vi "Run Process And Alg.vi"(7 "Process":bool, 8 "error in (no error)":errorcluster, 9 "CheckDist":bool, 10 "ROIList":string[][](array[string]), 11 "Image":T2(plugin-control)) -> (0 "Result Arr":T1(array[cluster]), 1 "DetectOut":variant[](array[variant]), 2 "ALLResultOut":string[][](array[string]), 3 "AlgOut":i32[](array[numeric]), 4 "error out":errorcluster)   [LabVIEW 2019]
uses:
  a08a38d4-8fb3-4640-b0fd-20f744aeac5c.vi
  1e835489-0bb4-467e-a464-32fccfa39e30.vi
  <vilib>/JDP Science/JSONtext/JSON text to Variant.vi
  Main UI/Glb/Main_UI Gb.vi
panel:
  out "x-y":u32
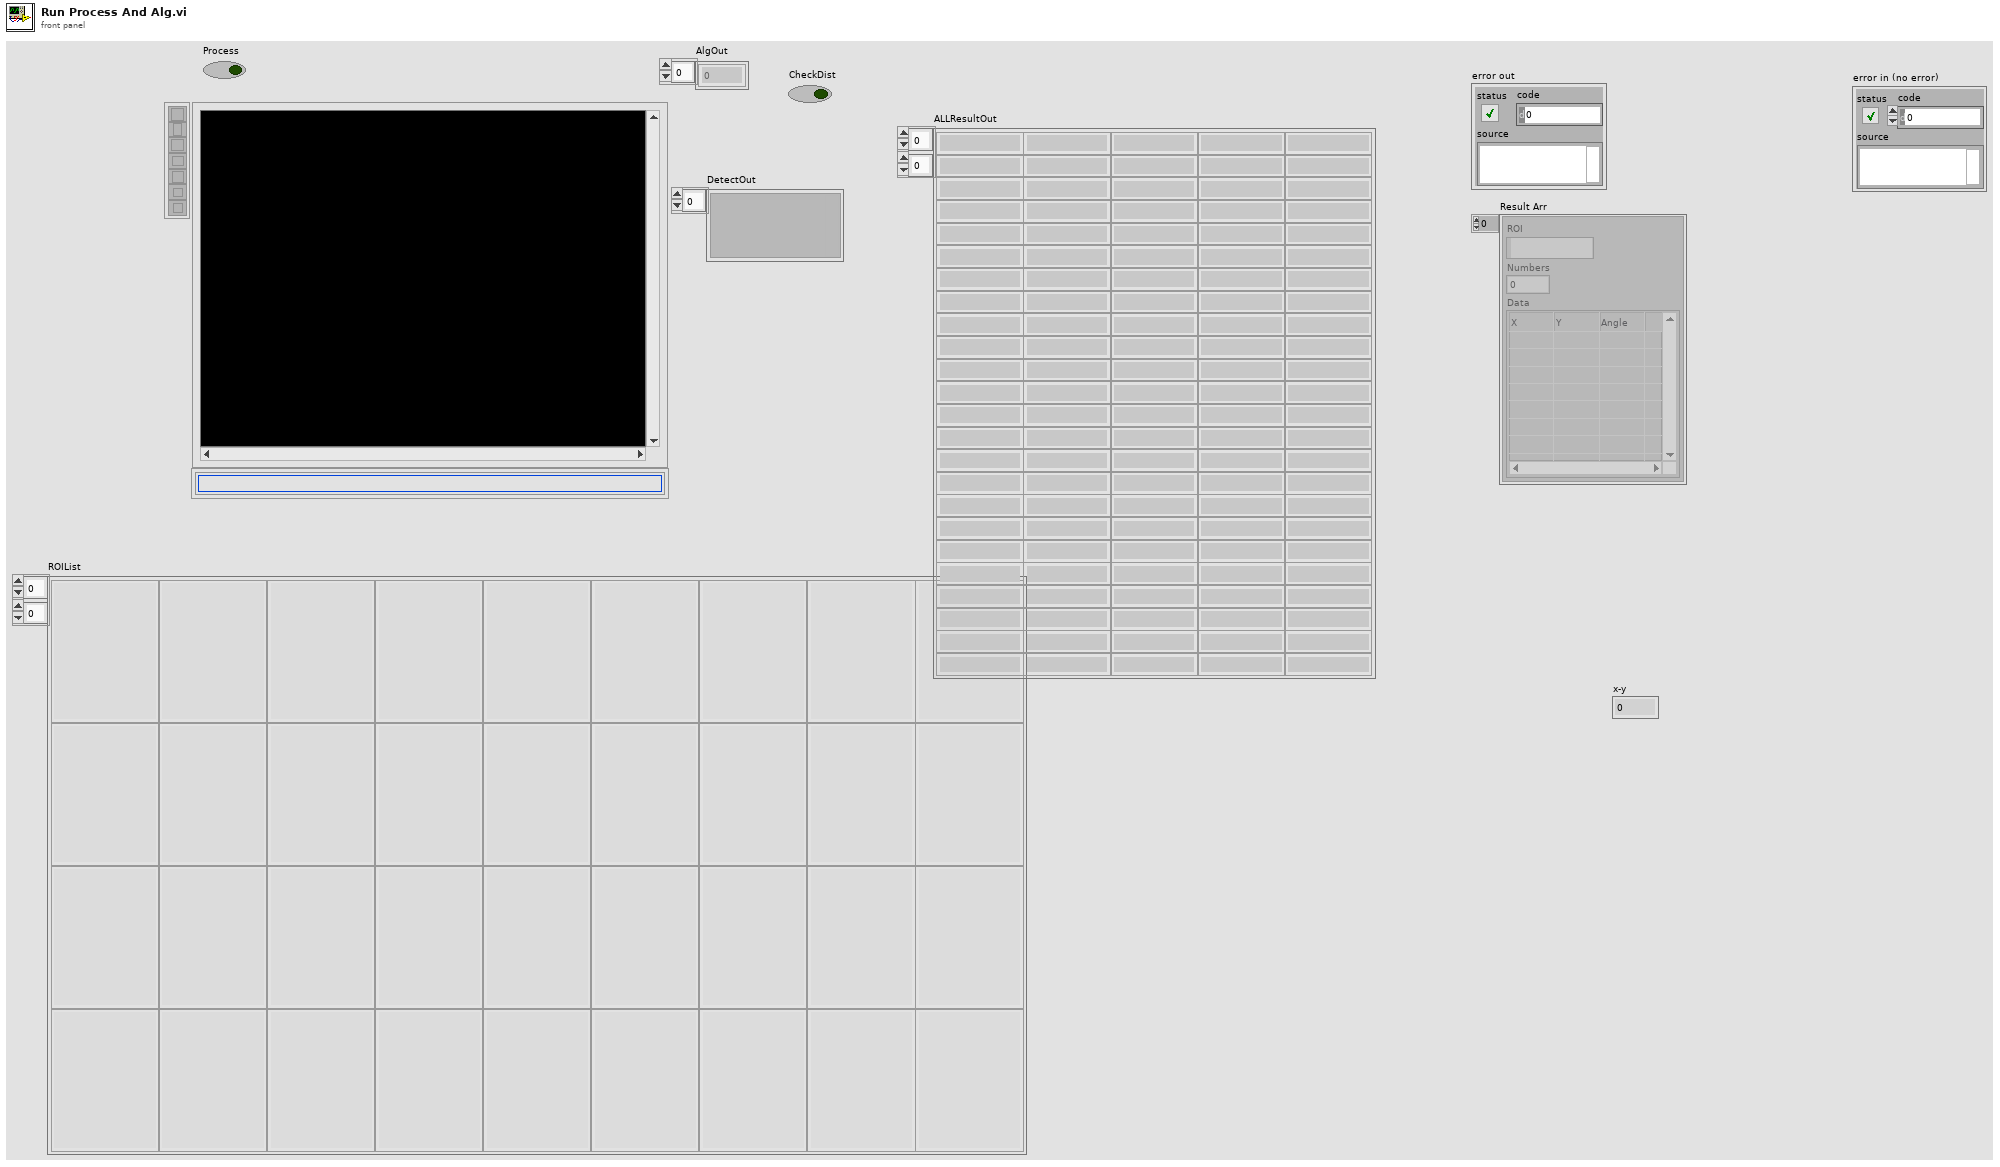
[diagram p1: front panel]
types:
  T1 = cluster{"ROI":string, "Numbers":i32, "Data":string[][]}[]
  T2 = typedef "IMAQ Image.ctl" = refnum<image>
  T3 = enum16{"Init", "Grab", "Get All", "Close", "Set Camera"}
  T4 = typedef "IMAQdx.ctl" = refnum<k21>
  T5 = cluster{"Desired Font (Application)":enum16{"User-specified Font", "Application Font", "System Font", "Dialog Font"}, "[User-specified Font]":cluster{"Font Name":string, "Size":i16, "Strikeout?":bool, "Italic?":bool, "Underline?":bool, "Outline?":bool, "Shadow?":bool, "Bold?":bool, "Rotation Angle":dbl}, "Horizontal Alignment":i16, "Vertical Alignment":i16}
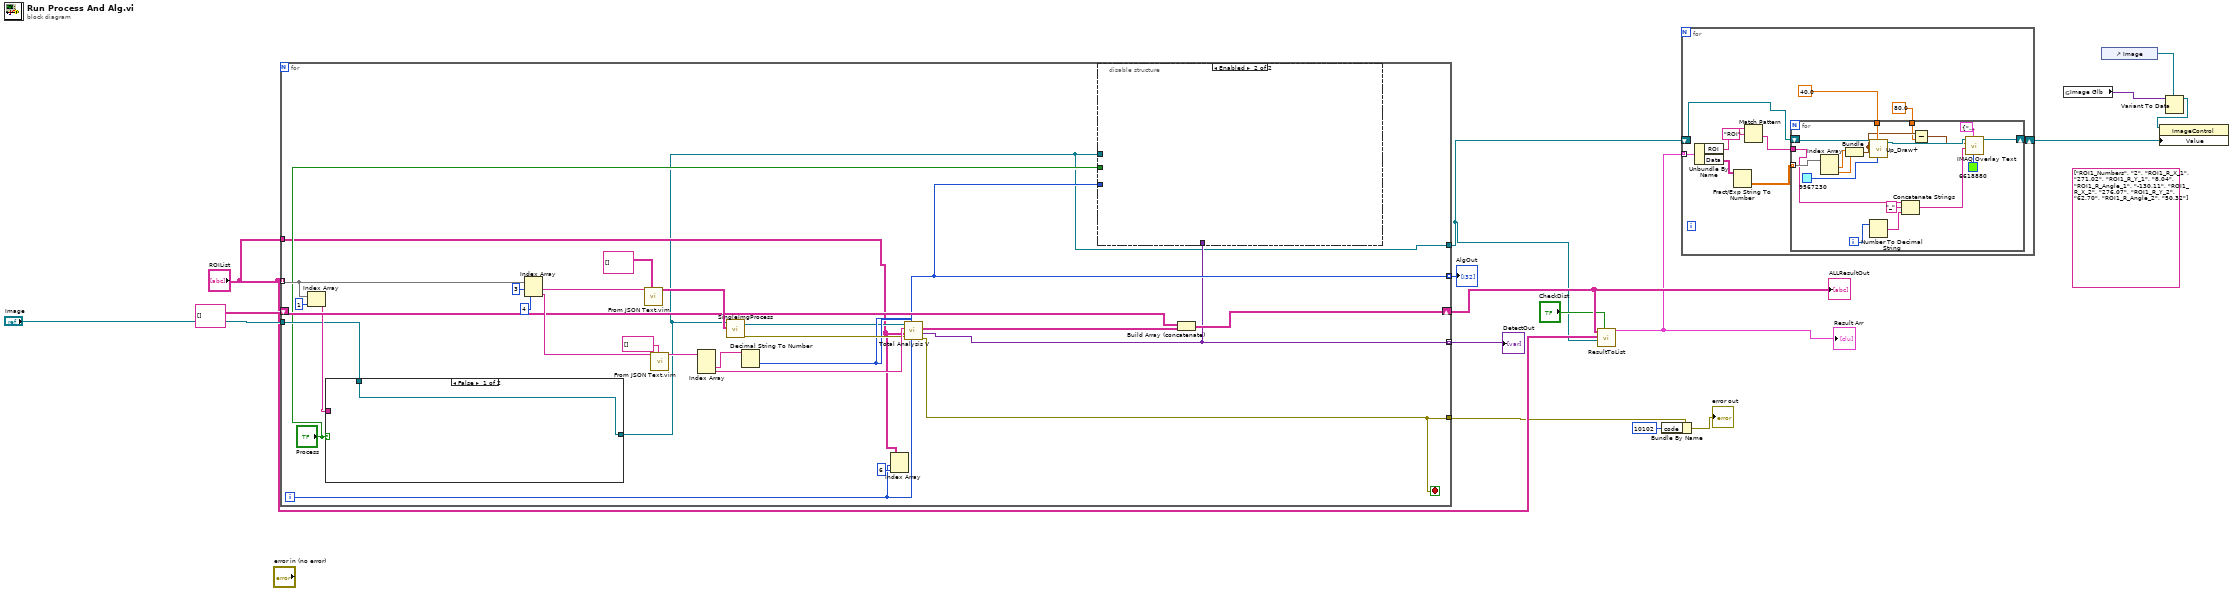
[diagram p0: block diagram]
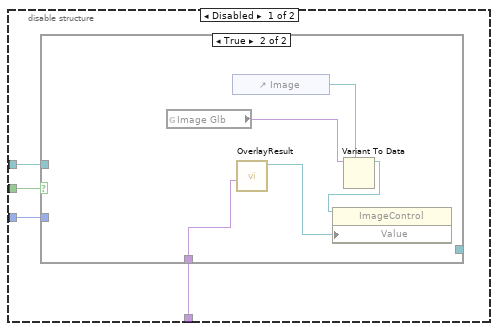
[diagram p2: hidden frame]
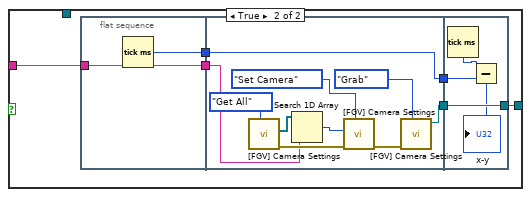
[diagram p4: hidden frame]
diagram:
  (unwired) string[][] [["ROI1_Numbers", "2"], ["ROI1_R_X_1", "271.02"], ["ROI1_R_Y_1", "8.04"], ["ROI1_R_Angle_1", "-130.11"], ["ROI1_R_X_2", "276.07"], ["ROI1_R_Y_2", "62.70"], ["ROI1_R_Angle_2", "50.32"]] ("ResultOut 2")
  n1 = for {
    tunnel: "ROIList" -> [w29] mode=indexing
    tunnel: "Image" -> [w26]
    shift-right: [w33] -> w13
    shift-left: string[][] [] -> [w32]
    tunnel: [w24] -> w3 mode=indexing
    tunnel: [w25] -> w14 mode=indexing
    tunnel: "ROIList" -> [w19]
    tunnel: [w18] -> w6
    tunnel: [w17] -> w1
    i -> [w21]
    stop <- w18 stop-if-true
    n2 = Index Array(array=w29, index=1) -> (element=w27:string)
    n3 = case shown="False" "Process" {
      tunnel: w27 -> [_ w60]
      tunnel: [w54 w59] -> w17
      tunnel: w26 -> [w54 _]
      frame False {
      }
      frame True {
        n4 = flat-sequence {
          tunnel: w60 -> [w62]
          tunnel: [w62] -> w58
          tunnel: [w61] -> w56
          tunnel: w58 -> [w65]
          tunnel: [w64] -> w57
          tunnel: w56 -> [w63]
          tunnel: [w63] -> w55
          tunnel: [w76] -> w59
          tunnel: w57 -> [w76]
          tunnel: w55 -> [w74]
          frame #0 {
            n5 = Tick Count (ms)() -> (millisecond timer value=w61:u32)
          }
          frame #1 {
            n6 = call "[FGV] Camera Settings.vi"("Action"=T3."Get All") -> ("error out"=w68:errorcluster, "Camera Interface Name"=w71:T4[])  [unwired: 8 in, 1 out]
            n7 = Search 1D Array(1D array=w71, element=w65) -> (index of element=w69:i32)  [unwired: 1 in]
            n8 = call "[FGV] Camera Settings.vi"("Action"=T3."Set Camera", "error in (no error)"=w68, "Value"=w69) -> ("error out"=w66:errorcluster)  [unwired: 6 in, 2 out]
            n9 = call "[FGV] Camera Settings.vi"("Action"=T3."Grab", "error in (no error)"=w66) -> ("Image Out"=w64:T2)  [unwired: 7 in, 2 out]
          }
          frame #2 {
            n10 = Tick Count (ms)() -> (millisecond timer value=w75:u32)
            n11 = Subtract(x=w75, y=w74) -> (x-y=→"x-y":u32)
          }
        }
      }
    }
    n12 = Index Array(array=w29, index #1=3 ("index"), index #2=4 ("index")) -> (element #1=w41:string, element #2=w38:string)
    n13 = call "From JSON Text.vim"("Data Type and Default Value"=string[][] [], "JSON"=w41) -> ("Data out"=w37:string[][])  [unwired: 8 in, 1 out]
    n14 = call "From JSON Text.vim"("Data Type and Default Value"=string[] [], "JSON"=w38) -> ("Data out"=w36:string[])  [unwired: 8 in, 1 out]
    n15 = Index Array(array=w36) -> (element #2=w34:string, element #3=w35:string)  [unwired: 3 in, 1 out]
    n16 = call "SingleImgProcess.vi"("Process List"=w37, "Refnum in"=w17) -> ("error out"=w31:errorcluster, "ImgOut"=w22:T2)  [unwired: 8 in]
    n17 = Decimal String To Number(string=w34) -> (number=w25:i32)  [unwired: 2 in, 1 out]
    n18 = Index Array(array=w19, index (row)=w21, index (col)=6 ("disabled index (col)")) -> ()  [unwired: 1 out]
    n19 = call "Total Analysis V.vi"("ROIIndex"=w21, "Algorithm"=w25, "error in"=w31, "ROIList"=w19, "AlgParameter"=w35, "Img in"=w22) -> ("error out"=w18:errorcluster, "DetectResult"=w24:variant, "ResultOut"=w20:string[][])  [unwired: 2 in, 1 out]
    n20 = disable-structure shown="Enabled" {
      disable-tunnel: w25 -> [w47 _]
      disable-tunnel: w24 -> [w46 _]
      disable-tunnel: "Process" -> [w45 _]
      disable-tunnel: w17 -> [w44 _]
      frame Disabled {
        n21 = case shown="True" w45 {
          tunnel: w47 -> [_ _]
          tunnel: w46 -> [_ w53]
          tunnel: w44 -> [w48 _]
          tunnel: [w48 _] -> _
          frame False {
          }
          frame True {
            n22 = global read "Main_UI Gb.vi" "Image Glb"() -> (w52:variant)
            n23 = control-ref of="Image"() -> (w51:refnum<vi>)
            n24 = call "OverlayResult.vi"("DectectResult"=w53) -> ("Image Out"=w49:T2)  [unwired: 10 in]
            n25 = Variant To Data(type=w51, Variant=w52) -> (data=w50:refnum<vi>)  [unwired: 1 in, 1 out]
            n26 = property class="ImageControl"(reference=w50, "Value"=w49) -> ()  [unwired: 1 in, 2 out]
          }
        }
      }
      frame Enabled {
      }
    }
    n27 = Build Array (concatenate)(w32, w20) -> (w33:string[][])
  }
  "ALLResultOut" <- w13
  "DetectOut" <- w3
  "AlgOut" <- w14
  n28 = call "ResultToList.vi"("CheckDist"="CheckDist", "Image In"=w1, "ROIList"="ROIList", "ALLResultOut"=w13) -> ("Result Arr"=w2:T1)  [unwired: 7 in]
  "Result Arr" <- w2
  n29 = Bundle By Name(cluster=w6, "code"=10102) -> (→"error out":errorcluster)
  n30 = for {
    shift-right: [w85] -> w8
    shift-left: w1 -> [w86]
    tunnel: w2 -> [w83] mode=indexing
    n31 = Unbundle By Name(w83) -> ("ROI"=w79:string, "Data"=w82:string[][])
    n32 = Fract/Exp String To Number(string=w82) -> (number=w81:dbl[][])  [unwired: 3 in, 1 out]
    n33 = Match Pattern(string=w79, regular expression="ROI") -> (after substring=w77:string)  [unwired: 1 in, 3 out]
    n34 = for {
      tunnel: 40.0 ("y") -> [w103]
      shift-right: [w95] -> w85
      shift-left: w86 -> [w104]
      tunnel: w81 -> [w101] mode=indexing
      tunnel: 80.0 ("y") -> [w97]
      tunnel: w77 -> [w92]
      i -> [w91]
      n35 = Index Array(array=w101) -> (element #1=w100:dbl, element #2=w99:dbl)  [unwired: 2 in]
      n36 = Bundle(w100, w99) -> (w98:cluster{dbl, dbl})  [unwired: 1 in]
      n37 = Number To Decimal String(number=w91) -> (decimal integer string=w90:string)  [unwired: 1 in]
      n38 = call "Up_Draw+.vi"("Color"=u32 9567230, "y"=w103, "Center"=w98, "Image"=w104) -> ("Image Out"=w96:T2)  [unwired: 7 in]
      n39 = Concatenate Strings(w92, "_" ("string"), w90) -> (w88:string)
      n40 = Subtract(x=w98, y=w97) -> (x-y=w87:cluster{dbl, dbl})
      n41 = call "IMAQ Overlay Text"("Text Color (black)"=u32 6618880, "Font, Size & Style"=T5 {"Desired Font (Application)"=enum."User-specified Font", "[User-specified Font]"={"Font Name"="", "Size"=48, "Strikeout?"=FALSE, "Italic?"=FALSE, "Underline?"=FALSE, "Outline?"=FALSE, "Shadow?"=FALSE, "Bold?"=FALSE, "Rotation Angle"=0.0}, "Horizontal Alignment"=1, "Vertical Alignment"=0}, "String"=w88, "Origin"=w87, "Image"=w96) -> ("Image Out"=w95:T2)  [unwired: 5 in, 1 out]
    }
  }
  n42 = global read "Main_UI Gb.vi" "Image Glb"() -> (w9:variant)
  n43 = control-ref of="Image"() -> (w10:refnum<vi>)
  n44 = Variant To Data(type=w10, Variant=w9) -> (data=w11:refnum<vi>)  [unwired: 1 in, 1 out]
  n45 = property class="ImageControl"(reference=w11, "Value"=w8) -> ()  [unwired: 1 in, 2 out]
